vi "PLC.AddProdComp.vi"(7 "Idx":i32, 8 "error in":errorcluster, 11 "Data_in":T1={"Status"={"Idx"=0, "ConnRef"=0, "State"=enum."Off", "LiveBitTimer"=timestamp(0 s since 1904-01-01)}, "Sets"={"Enable"=FALSE, "IP"="", "Rack"=0, "Slot"=0, "LifeBitTimer_s"=0.0, "DataBlockAddr_PCStatus"=0, "DataBlockAddr_PLCStatus"=1, "DataBlockAddr_PLCNewData"=[], "DataBlockSize_PLCNewData"=[], "DataBlockAddr_PLCChangeOver"=[], "DataBlockSize_PLCChangeOver"=[], "DataBlockAddr_PCChangeOver"=[], "DataBlockSize_PCChangeOver"=[], "DataBlockAddr_PLCCheckStatus"=[], "DataBlockSize_PLCCheckStatus"=[], "DataBlockAddr_PCCheckStatus"=[], "DataBlockSize_PCCheckStatus"=[]}, "PCstatus"={"General"={"LifeBit"=FALSE, "DbRun"=FALSE}, "Stations"=[]}, "PLCstatus"={"General"={"LifeBit"=FALSE}, "Slots"=[]}, "PLCValues"=[]} {"PLCValues"."Values" format="%.3f"}) -> (0 "error out":errorcluster, 3 "Data_out":T1={"Status"={"Idx"=0, "ConnRef"=0, "State"=enum."Off", "LiveBitTimer"=timestamp(0 s since 1904-01-01)}, "Sets"={"Enable"=FALSE, "IP"="", "Rack"=0, "Slot"=0, "LifeBitTimer_s"=0.0, "DataBlockAddr_PCStatus"=0, "DataBlockAddr_PLCStatus"=1, "DataBlockAddr_PLCNewData"=[], "DataBlockSize_PLCNewData"=[], "DataBlockAddr_PLCChangeOver"=[], "DataBlockSize_PLCChangeOver"=[], "DataBlockAddr_PCChangeOver"=[], "DataBlockSize_PCChangeOver"=[], "DataBlockAddr_PLCCheckStatus"=[], "DataBlockSize_PLCCheckStatus"=[], "DataBlockAddr_PCCheckStatus"=[], "DataBlockSize_PCCheckStatus"=[]}, "PCstatus"={"General"={"LifeBit"=FALSE, "DbRun"=FALSE}, "Stations"=[]}, "PLCstatus"={"General"={"LifeBit"=FALSE}, "Slots"=[]}, "PLCValues"=[]} {"PLCValues"."Values" format="%.3f"})   [LabVIEW 2016]
doc: "Get test results (measurement values) from PLC and save to database\n\nWabco 2017 All right reserved\nAuthor: maciej.szupienko@wabco-auto.com"
uses:
  PLC.Data.Sets.ctl
  PLC.State.ctl
  PLC.Data.Status.ctl
  PLC.Data.ctl
  LowLevel/PLC.DataBlock.PCstatus.ctl
  LowLevel/PLC.DataBlock.PLCstatus.ctl
  LowLevel/PLC.DataBlock.PLCvalues.ctl
  LowLevel/PLC.DataBlock.PLCstatus.Station.ctl
  LowLevel/PLC.DataBlock.PLCstatus.General.ctl
  LowLevel/PLC.DataBlock.PCstatus.Station.ctl
  LowLevel/PLC.DataBlock.PCstatus.General.ctl
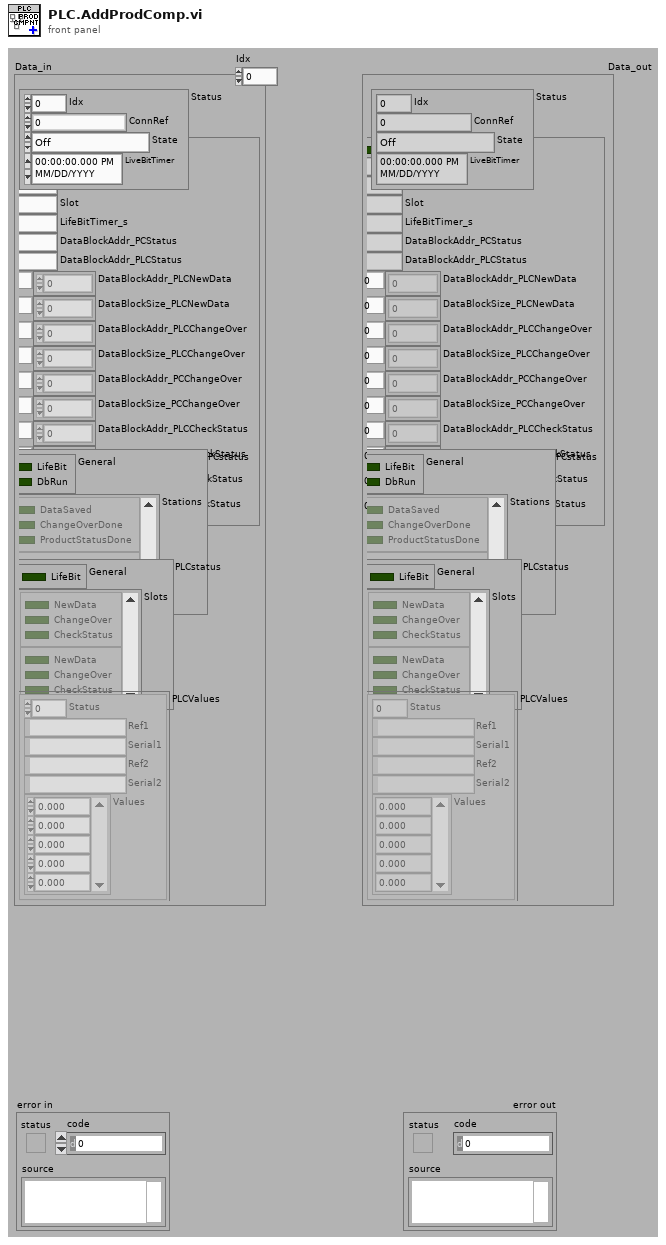
[diagram p1: front panel]
types:
  T1 = typedef "PLC.Data.ctl" = cluster{"Status":T2, "Sets":T4, "PCstatus":T5, "PLCstatus":T8, "PLCValues":T11[]}
  T2 = typedef "PLC.Data.Status.ctl" = cluster{"Idx":i32, "ConnRef":u64, "State":T3, "LiveBitTimer":timestamp}
  T3 = typedef "PLC.State.ctl" = enum32{"Off", "Error", "Idle", "Run"}
  T4 = typedef "PLC.Data.Sets.ctl" = cluster{"Enable":bool, "IP":string, "Rack":i32, "Slot":i32, "LifeBitTimer_s":dbl, "DataBlockAddr_PCStatus":i32, "DataBlockAddr_PLCStatus":i32, "DataBlockAddr_PLCNewData":i32[], "DataBlockSize_PLCNewData":i32[], "DataBlockAddr_PLCChangeOver":i32[], "DataBlockSize_PLCChangeOver":i32[], "DataBlockAddr_PCChangeOver":i32[], "DataBlockSize_PCChangeOver":i32[], "DataBlockAddr_PLCCheckStatus":i32[], "DataBlockSize_PLCCheckStatus":i32[], "DataBlockAddr_PCCheckStatus":i32[], "DataBlockSize_PCCheckStatus":i32[]}
  T5 = typedef "PLC.DataBlock.PCstatus.ctl" = cluster{"General":T6, "Stations":T7[]}
  T6 = typedef "PLC.DataBlock.PCstatus.General.ctl" = cluster{"LifeBit":bool, "DbRun":bool}
  T7 = typedef "PLC.DataBlock.PCstatus.Station.ctl" = cluster{"DataSaved":bool, "ChangeOverDone":bool, "ProductStatusDone":bool}
  T8 = typedef "PLC.DataBlock.PLCstatus.ctl" = cluster{"General":T9, "Slots":T10[]}
  T9 = typedef "PLC.DataBlock.PLCstatus.General.ctl" = cluster{"LifeBit":bool}
  T10 = typedef "PLC.DataBlock.PLCstatus.Slot.ctl" = cluster{"NewData":bool, "ChangeOver":bool, "CheckStatus":bool}
  T11 = typedef "PLC.DataBlock.PLCvalues.ctl" = cluster{"Status":u8, "Ref1":string, "Serial1":string, "Ref2":string, "Serial2":string, "Values":sgl[]}
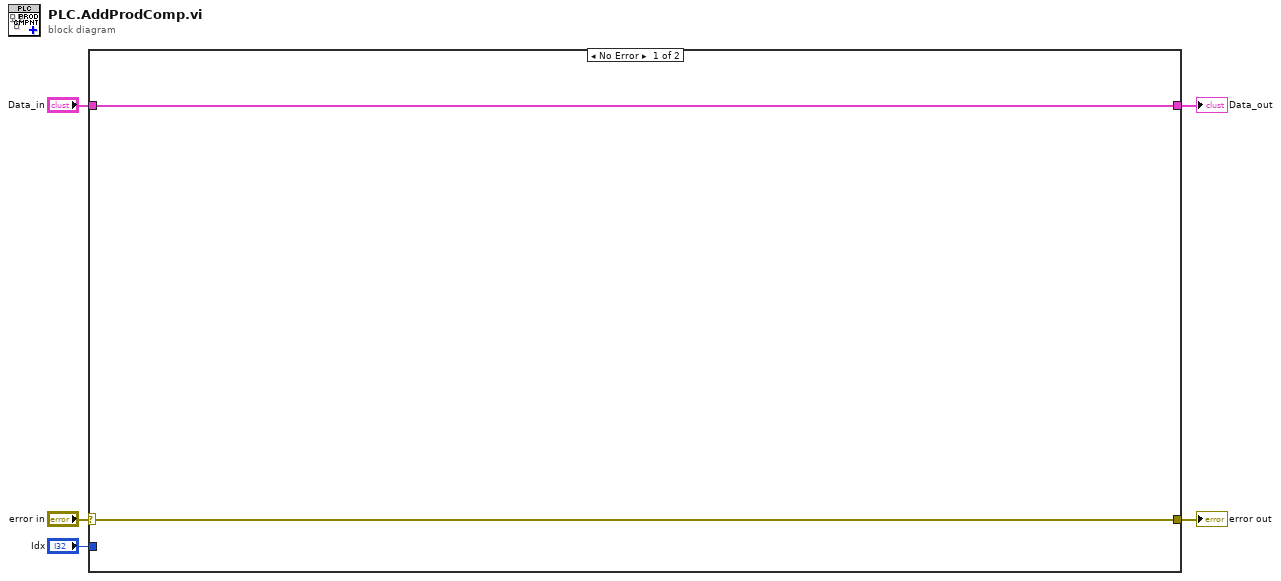
[diagram p0: block diagram]
diagram:
  n1 = case shown="No Error" "error in" {
    selector: "error in" -> [w6 w9]
    tunnel: [w6 w9] -> w2
    tunnel: "Data_in" -> [w7 w8]
    tunnel: [w7 w8] -> w4
    tunnel: "Idx" -> [_ _]
    frame No Error {
    }
    frame Error {
    }
  }
  "error out" <- w2
  "Data_out" <- w4
